vi "TrainModel.vi"(8 "error in (no error)":errorcluster, 9 "Finished":bool, 10 "Robot":refnum<class "Robot.lvclass">, 11 "Navigation in":refnum<class "Navigation.lvclass">) -> (0 "error out":errorcluster, 3 "Navigation out":refnum<class "Navigation.lvclass">)   [LabVIEW 2023, in "Navigation.lvclass"]
uses:
  Navigation.lvclass
  Robot_class/Robot.lvclass
  C:/Users/ebert/Desktop/roboime/SSL_AI/Object_class/Object.lvclass
  Robot_class/Robot.lvclass/Robot.ctl
  Object_class/Object.lvclass/Object.ctl
  Controls/RobotModel.ctl
  Robot_class/Read id.vi
  Object_class/Read position(x,y).vi
  Robot_class/Read est_v_norm.vi
  Robot_class/Read est_v_tang.vi
  Robot_class/Read v_norm.vi
  Robot_class/Read v_tang.vi
  Utilities_class/Utilities.lvclass
panel:
  in  "RobotModelFolder":string
  out "error out 2":errorcluster
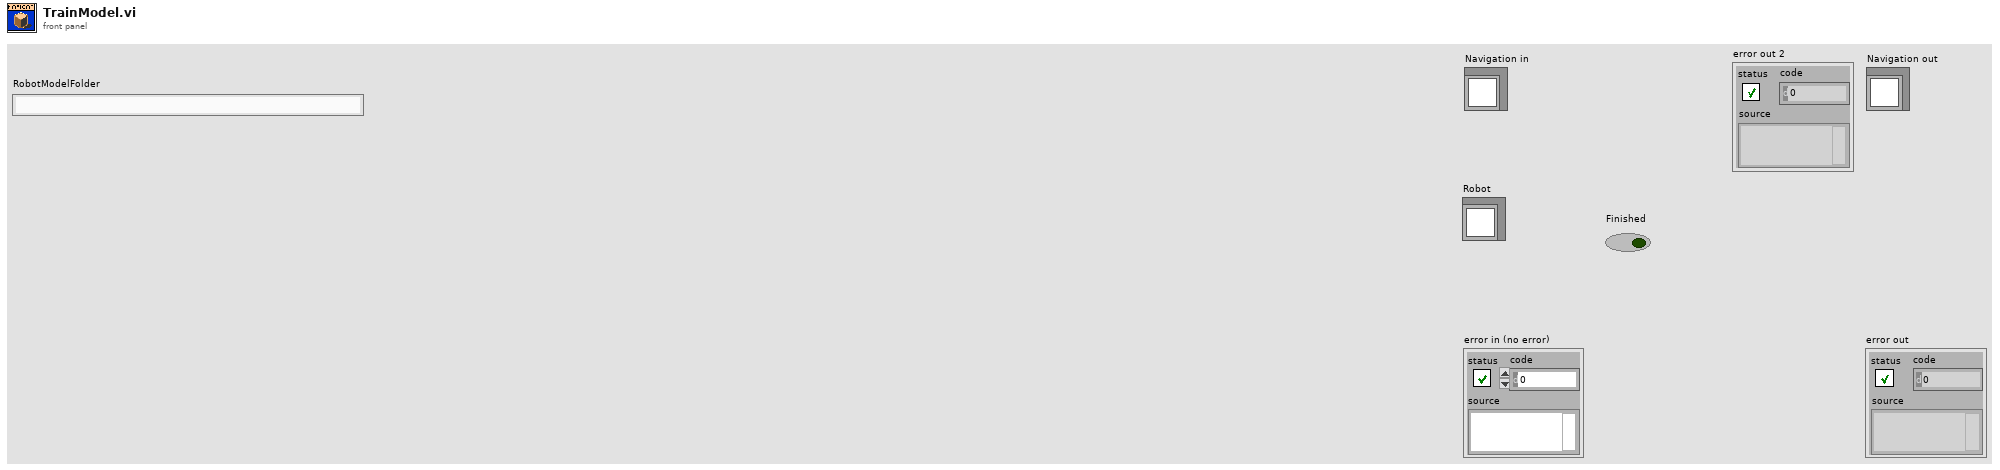
[diagram p1: front panel]
types:
  T1 = typedef "RobotModel.ctl" = cluster{"V0":dbl, "Vf":dbl, "Dist":dbl, "dt":dbl, "P1":dbl[], "P2":dbl[], "V_sent":dbl, "sampleNumber":i32, "triple_id":i32, "consideredSamples":dbl[]}
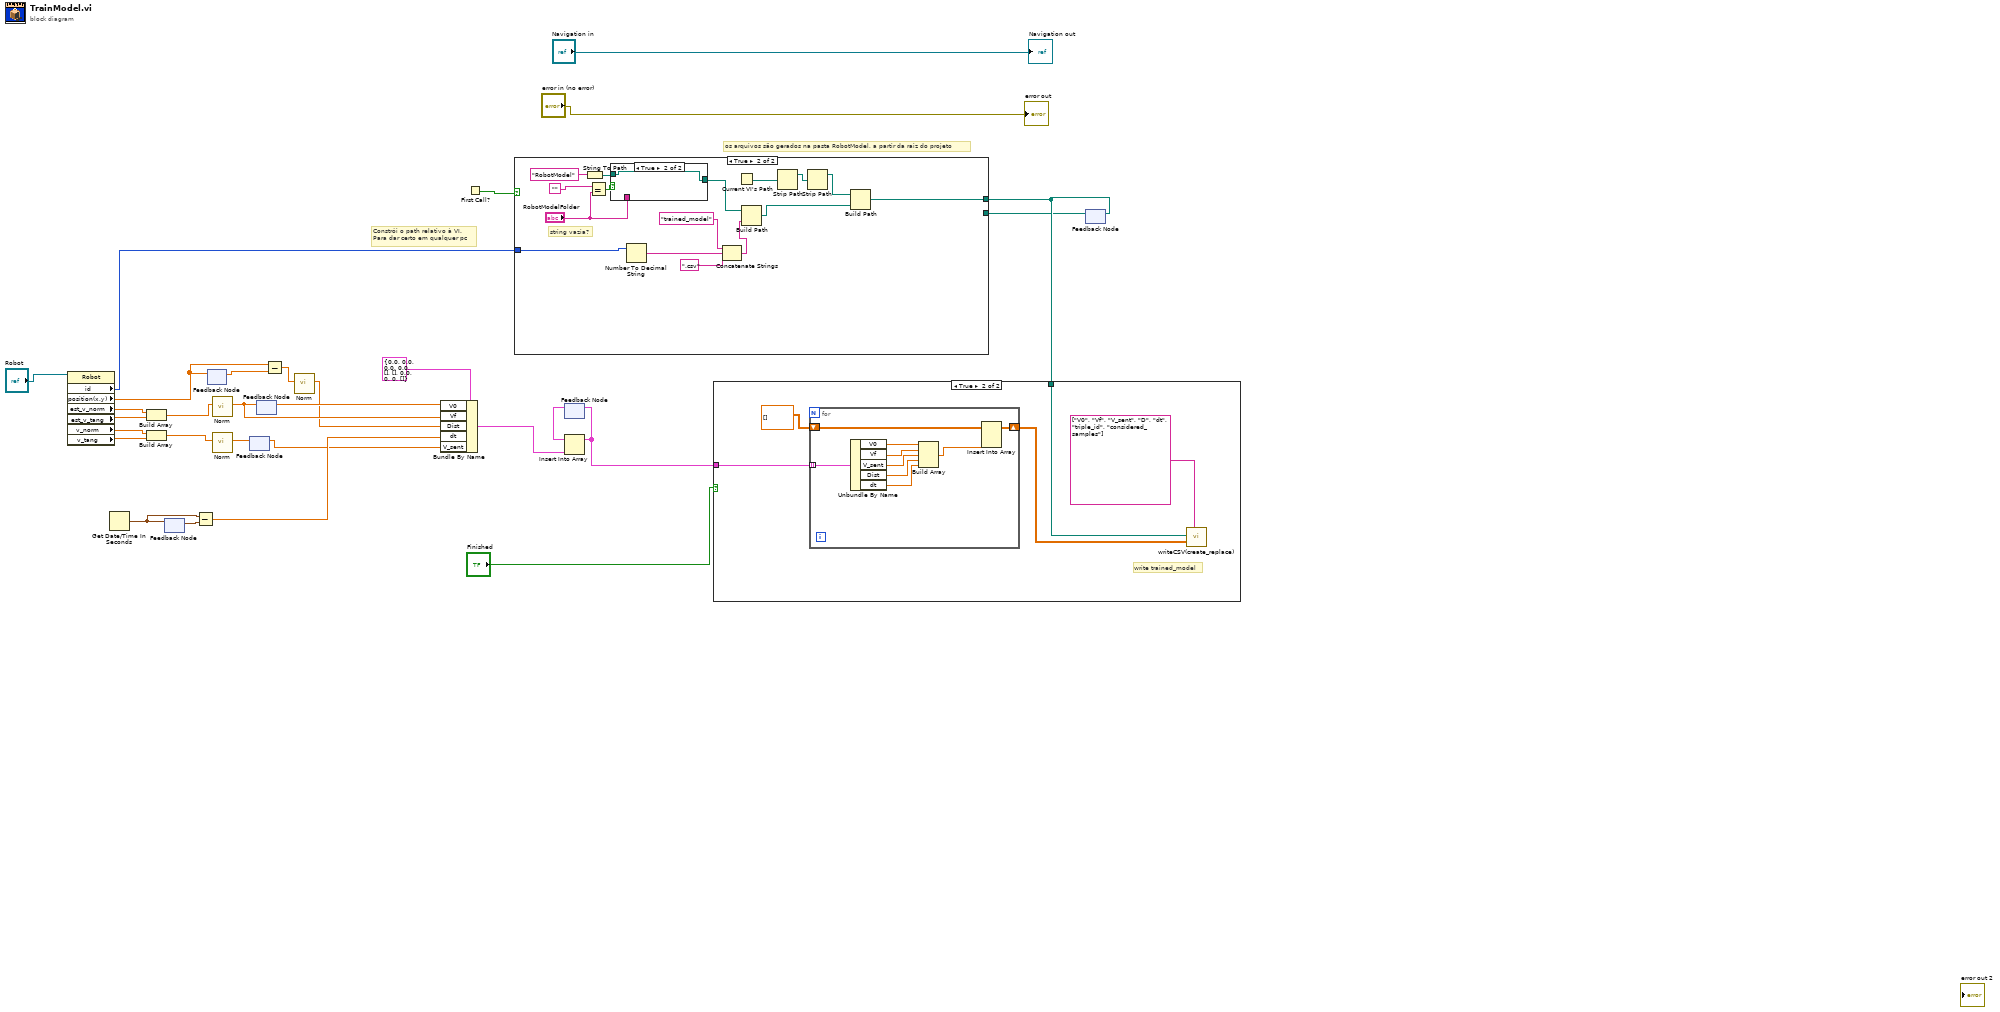
[diagram p0: block diagram]
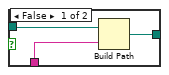
[diagram p4: hidden frame]
diagram:
  # "os arquivos são gerados na pasta RobotModel, a partir da raiz do projeto"
  # "Constrói o path relativo à VI.\nPara dar certo em qualquer pc"
  n1 = property class="Robot"(reference="Robot") -> ("id"=w5:i32, "position(x,y)"=w13:dbl[], "est_v_norm"=w23:dbl, "est_v_tang"=w22:dbl, "v_norm"=w21:dbl, "v_tang"=w20:dbl)  [unwired: 1 in, 2 out]
  n2 = Get Date/Time In Seconds() -> (seconds since 1Jan1904=w8:timestamp)
  n3 = Build Array(w23, w22) -> (w19:dbl[])
  n4 = Build Array(w21, w20) -> (w18:dbl[])
  n5 = feedback #1() -> (w9:timestamp)  [unwired: 1 in]
  n6 = feedback-in #1(w8) -> ()
  n7 = Subtract(x=w8, y=w9) -> (x-y=w7:dbl)
  n8 = feedback #2() -> (w12:dbl[])  [unwired: 1 in]
  n9 = feedback-in #2(w13) -> ()
  n10 = call "Norm.vi"("2D vector"=w19) -> ("Modulo"=w14:dbl)  [unwired: 8 in, 2 out]
  n11 = call "Norm.vi"("2D vector"=w18) -> ("Modulo"=w17:dbl)  [unwired: 8 in, 2 out]
  n12 = feedback-in #3(w17) -> ()
  n13 = feedback #3() -> (w6:dbl)  [unwired: 1 in]
  n14 = feedback #4() -> (w15:dbl)  [unwired: 1 in]
  n15 = feedback-in #4(w14) -> ()
  n16 = Subtract(x=w13, y=w12) -> (x-y=w11:dbl[])
  n17 = call "Norm.vi"("2D vector"=w11) -> ("Modulo"=w10:dbl)  [unwired: 8 in, 2 out]
  n18 = Bundle By Name(cluster=T1 {"V0"=0.0, "Vf"=0.0, "Dist"=0.0, "dt"=0.0, "P1"=[], "P2"=[], "V_sent"=0.0, "sampleNumber"=0, "triple_id"=0, "consideredSamples"=[]} ("input cluster"), "V0"=w15, "Vf"=w14, "Dist"=w10, "dt"=w7, "V_sent"=w6) -> (w4:T1)
  n19 = First Call?() -> (First Call?: T/F=w25:bool)
  n20 = feedback #5() -> (w3:T1[])  [unwired: 1 in]
  n21 = Insert Into Array(array=w3, new element=w4) -> (w2:T1[])  [unwired: 1 in]
  n22 = feedback-in #5(w2) -> ()
  n23 = feedback #6() -> (w26:path)  [unwired: 1 in]
  n24 = case shown="True" w25 {
    tunnel: [w30 w44] -> w27
    tunnel: w26 -> [w30 _]
    tunnel: w5 -> [_ w35]
    frame False {
      # "só precisa calcular o path na 1° iteração"
    }
    frame True {
      # "string vazia?"
      n25 = String To Path(string="RobotModel" ("name or relative path")) -> (path=w38:path)
      n26 = Equal?(x="", y="RobotModelFolder") -> (x = y?=w42:bool)
      n27 = case shown="True" w42 {
        tunnel: "RobotModelFolder" -> [w49 _]
        tunnel: [w48 w50] -> w37
        tunnel: w38 -> [w47 w50]
        frame False {
          n28 = Build Path(base path=w47, name or relative path=w49) -> (appended path=w48:path)
        }
        frame True {
        }
      }
      n29 = Number To Decimal String(number=w35) -> (decimal integer string=w33:string)  [unwired: 1 in]
      n30 = Concatenate Strings("trained_model" ("name or relative path"), w33, ".csv" ("name or relative path")) -> (w32:string)
      n31 = Current VI's Path() -> (path=w46:path)
      n32 = Build Path(base path=w37, name or relative path=w32) -> (appended path=w43:path)
      n33 = Strip Path(path=w46) -> (stripped path=w45:path)  [unwired: 1 out]
      n34 = Strip Path(path=w45) -> (stripped path=w36:path)  [unwired: 1 out]
      n35 = Build Path(base path=w36, name or relative path=w43) -> (appended path=w44:path)
    }
  }
  n36 = case shown="True" "Finished" {
    tunnel: w27 -> [_ w55]
    tunnel: w2 -> [_ w51]
    frame False {
    }
    frame True {
      # "write trained_model"
      n37 = for {
        shift-right: [w63] -> w53
        shift-left: dbl[][] [] ("Array") -> [w64]
        tunnel: w51 -> [w56] mode=indexing
        n38 = Unbundle By Name(w56) -> ("V0"=w62:dbl, "Vf"=w61:dbl, "V_sent"=w60:dbl, "Dist"=w59:dbl, "dt"=w58:dbl)
        n39 = Build Array(w62, w61, w60, w59, w58) -> (w57:dbl[])
        n40 = Insert Into Array(array=w64, new element=w57) -> (w63:dbl[][])  [unwired: 2 in]
      }
      n41 = call "writeCSV(create_replace).vi"("Header"=string[] ["V0", "Vf", "V_sent", "D", "dt", "triple_id", "considered_samples"] ("trained_model_header (default)"), "Array"=w53, "file path (use dialog)"=w55) -> ()  [unwired: 7 in, 2 out]
    }
  }
  n42 = feedback-in #6(w27) -> ()
  "error out" <- "error in (no error)"
  "Navigation out" <- "Navigation in"
